vi "Controle Position PilMOT.vi"() -> ()   [LabVIEW 2012]
panel:
  in  "NumeroParametre_E":u16
  in  "REF 2":bool
  out "Valeur_L":i32
  out "Numero_L":u16
  out "Messages_L":u32
  in  "REF":bool
  in  "Axe1_Vitesse":u16
  in  "Axe1_CoteAAtteindre":i32
  in  "MVT":bool
  out "Acquittement":u16
  in  "Prise Origine":bool
  in  "Gestion Application":bool
  in  "stop":bool
  in  "startSens-":bool
  in  "startSens+":bool
  out "Message Axe n°1":u16 format="%b"
  out "Position Théorique Axe n°1":i32
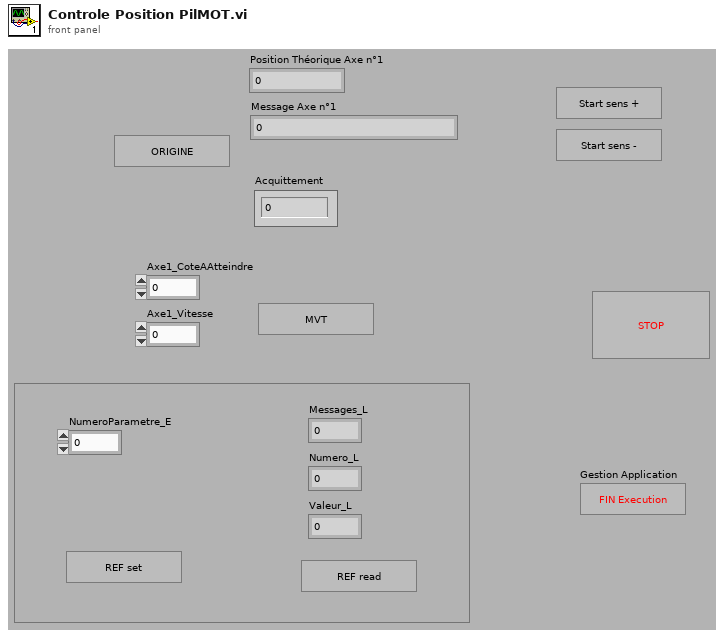
[diagram p1: front panel]
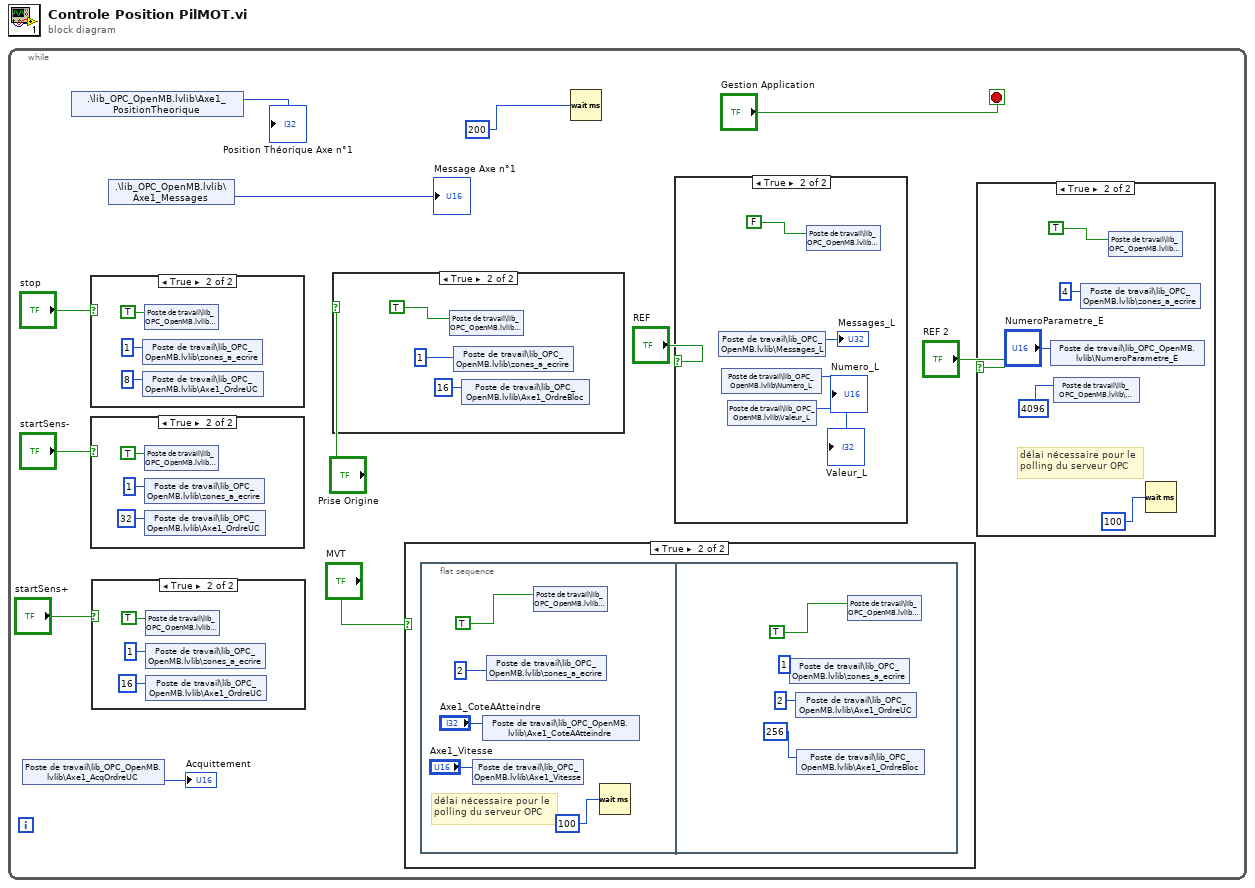
[diagram p0: block diagram]
diagram:
  n1 = while {
    stop <- "Gestion Application" stop-if-true
    n2 = shared-variable "Poste de travail\\lib_OPC_OpenMB.lvlib\\Axe1_AcqOrdreUC"() -> (→"Acquittement":u16)  [unwired: 1 in, 1 out]
    n3 = shared-variable ".\\lib_OPC_OpenMB.lvlib\\Axe1_PositionTheorique"() -> (→"Position Théorique Axe n°1":i32)  [unwired: 1 in, 1 out]
    n4 = case shown="True" "stop" {
      frame False {
      }
      frame True {
        n5 = shared-variable "Poste de travail\\lib_OPC_OpenMB.lvlib\\zones_a_ecrire"(u16 1 ("zones_a_ecrire")) -> ()  [unwired: 1 in, 1 out]
        n6 = shared-variable "Poste de travail\\lib_OPC_OpenMB.lvlib\\Axe1_OrdreUC"(u16 8 ("Axe1_OrdreUC")) -> ()  [unwired: 1 in, 1 out]
        n7 = shared-variable "Poste de travail\\lib_OPC_OpenMB.lvlib\\ecrire"(TRUE ("ecrire")) -> ()  [unwired: 1 in, 1 out]
      }
    }
    n8 = case shown="True" "startSens-" {
      frame False {
      }
      frame True {
        n9 = shared-variable "Poste de travail\\lib_OPC_OpenMB.lvlib\\ecrire"(TRUE ("ecrire")) -> ()  [unwired: 1 in, 1 out]
        n10 = shared-variable "Poste de travail\\lib_OPC_OpenMB.lvlib\\zones_a_ecrire"(u16 1 ("zones_a_ecrire")) -> ()  [unwired: 1 in, 1 out]
        n11 = shared-variable "Poste de travail\\lib_OPC_OpenMB.lvlib\\Axe1_OrdreUC"(u16 32 ("Axe1_OrdreUC")) -> ()  [unwired: 1 in, 1 out]
      }
    }
    n12 = case shown="True" "startSens+" {
      frame False {
      }
      frame True {
        n13 = shared-variable "Poste de travail\\lib_OPC_OpenMB.lvlib\\ecrire"(TRUE ("ecrire")) -> ()  [unwired: 1 in, 1 out]
        n14 = shared-variable "Poste de travail\\lib_OPC_OpenMB.lvlib\\zones_a_ecrire"(u16 1 ("zones_a_ecrire")) -> ()  [unwired: 1 in, 1 out]
        n15 = shared-variable "Poste de travail\\lib_OPC_OpenMB.lvlib\\Axe1_OrdreUC"(u16 16 ("Axe1_OrdreUC")) -> ()  [unwired: 1 in, 1 out]
      }
    }
    n16 = shared-variable ".\\lib_OPC_OpenMB.lvlib\\Axe1_Messages"() -> (→"Message Axe n°1":u16)  [unwired: 1 in, 1 out]
    n17 = case shown="True" "Prise Origine" {
      frame False {
      }
      frame True {
        n18 = shared-variable "Poste de travail\\lib_OPC_OpenMB.lvlib\\ecrire"(TRUE ("ecrire")) -> ()  [unwired: 1 in, 1 out]
        n19 = shared-variable "Poste de travail\\lib_OPC_OpenMB.lvlib\\zones_a_ecrire"(u16 1 ("zones_a_ecrire")) -> ()  [unwired: 1 in, 1 out]
        n20 = shared-variable "Poste de travail\\lib_OPC_OpenMB.lvlib\\Axe1_OrdreBloc"(u32 16 ("Axe1_OrdreBloc")) -> ()  [unwired: 1 in, 1 out]
      }
    }
    n21 = case shown="True" "MVT" {
      frame False {
      }
      frame True {
        n22 = flat-sequence {
          frame #0 {
            # "délai nécessaire pour le\npolling du serveur OPC"
            n23 = shared-variable "Poste de travail\\lib_OPC_OpenMB.lvlib\\Axe1_Vitesse"("Axe1_Vitesse") -> ()  [unwired: 1 in, 1 out]
            n24 = shared-variable "Poste de travail\\lib_OPC_OpenMB.lvlib\\Axe1_CoteAAtteindre"("Axe1_CoteAAtteindre") -> ()  [unwired: 1 in, 1 out]
            n25 = shared-variable "Poste de travail\\lib_OPC_OpenMB.lvlib\\zones_a_ecrire"(u16 2 ("zones_a_ecrire")) -> ()  [unwired: 1 in, 1 out]
            n26 = shared-variable "Poste de travail\\lib_OPC_OpenMB.lvlib\\ecrire"(TRUE ("ecrire")) -> ()  [unwired: 1 in, 1 out]
            n27 = Wait (ms)(milliseconds to wait=u32 100) -> ()  [unwired: 1 out]
          }
          frame #1 {
            n28 = shared-variable "Poste de travail\\lib_OPC_OpenMB.lvlib\\zones_a_ecrire"(u16 1 ("zones_a_ecrire")) -> ()  [unwired: 1 in, 1 out]
            n29 = shared-variable "Poste de travail\\lib_OPC_OpenMB.lvlib\\Axe1_OrdreUC"(u16 2 ("Axe1_OrdreUC")) -> ()  [unwired: 1 in, 1 out]
            n30 = shared-variable "Poste de travail\\lib_OPC_OpenMB.lvlib\\Axe1_OrdreBloc"(u32 256 ("Axe1_OrdreBloc")) -> ()  [unwired: 1 in, 1 out]
            n31 = shared-variable "Poste de travail\\lib_OPC_OpenMB.lvlib\\ecrire"(TRUE ("ecrire")) -> ()  [unwired: 1 in, 1 out]
          }
        }
      }
    }
    n32 = Wait (ms)(milliseconds to wait=u32 200) -> ()  [unwired: 1 out]
    n33 = case shown="True" "REF" {
      frame False {
      }
      frame True {
        n34 = shared-variable "Poste de travail\\lib_OPC_OpenMB.lvlib\\Messages_L"() -> (→"Messages_L":u32)  [unwired: 1 in, 1 out]
        n35 = shared-variable "Poste de travail\\lib_OPC_OpenMB.lvlib\\Numero_L"() -> (→"Numero_L":u16)  [unwired: 1 in, 1 out]
        n36 = shared-variable "Poste de travail\\lib_OPC_OpenMB.lvlib\\Valeur_L"() -> (→"Valeur_L":i32)  [unwired: 1 in, 1 out]
        n37 = shared-variable "Poste de travail\\lib_OPC_OpenMB.lvlib\\ecrire"(FALSE ("ecrire")) -> ()  [unwired: 1 in, 1 out]
      }
    }
    n38 = case shown="True" "REF 2" {
      frame False {
      }
      frame True {
        # "délai nécessaire pour le\npolling du serveur OPC"
        n39 = shared-variable "Poste de travail\\lib_OPC_OpenMB.lvlib\\NumeroParametre_E"("NumeroParametre_E") -> ()  [unwired: 1 in, 1 out]
        n40 = shared-variable "Poste de travail\\lib_OPC_OpenMB.lvlib\\Ordre_E"(u16 4096 ("Ordre")) -> ()  [unwired: 1 in, 1 out]
        n41 = shared-variable "Poste de travail\\lib_OPC_OpenMB.lvlib\\zones_a_ecrire"(u16 4 ("zones_a_ecrire")) -> ()  [unwired: 1 in, 1 out]
        n42 = shared-variable "Poste de travail\\lib_OPC_OpenMB.lvlib\\ecrire"(TRUE ("ecrire")) -> ()  [unwired: 1 in, 1 out]
        n43 = Wait (ms)(milliseconds to wait=u32 100) -> ()  [unwired: 1 out]
      }
    }
  }
